vi "MateChecker.vi"(10 "Turn":T1, 11 "Input Squares":T2[][](array[typedef])) -> (3 "Checkmate?":bool)   [LabVIEW 2019]
uses:
  #typedef_DataBase.ctl
  #typedef_SquareType.ctl
  #typedef_Color.ctl
  #typedef_Piece.ctl
  #typedef_PieceType.ctl
  #typedef_SquareLook.ctl
  #typedef_SpecialMoves.ctl
panel:
  out "?":u16[][](array[ring])
  in  "DataBase":T5
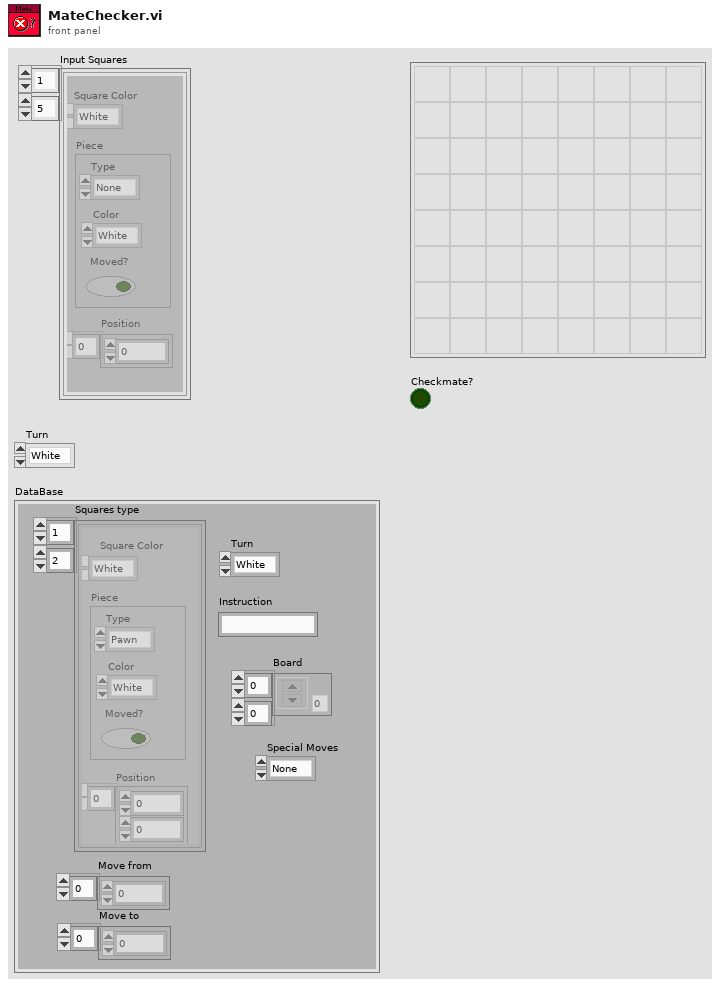
[diagram p1: front panel]
types:
  T1 = typedef "#typedef_Color.ctl" = enum16{"White", "Black"}
  T2 = typedef "#typedef_SquareType.ctl" = cluster{"Square Color":T1, "Position":i32[], "Piece":T3}
  T3 = typedef "#typedef_Piece.ctl" = cluster{"Type":T4, "Color":T1, "Moved?":bool}
  T4 = typedef "#typedef_PieceType.ctl" = enum16{"None", "Pawn", "Knight", "Bishop", "Rook", "Queen", "King"}
  T5 = typedef "#typedef_DataBase.ctl" = cluster{"Squares type":T2[][], "Turn":T1, "Move from":i32[], "Move to":i32[], "Instruction":string, "Board":T6[][], "Special Moves":T7}
  T6 = typedef "#typedef_SquareLook.ctl" = u16
  T7 = typedef "#typedef_SpecialMoves.ctl" = enum16{"None", "Last Square", "Beat in the Passage", "Short Castle", "Long Castle"}
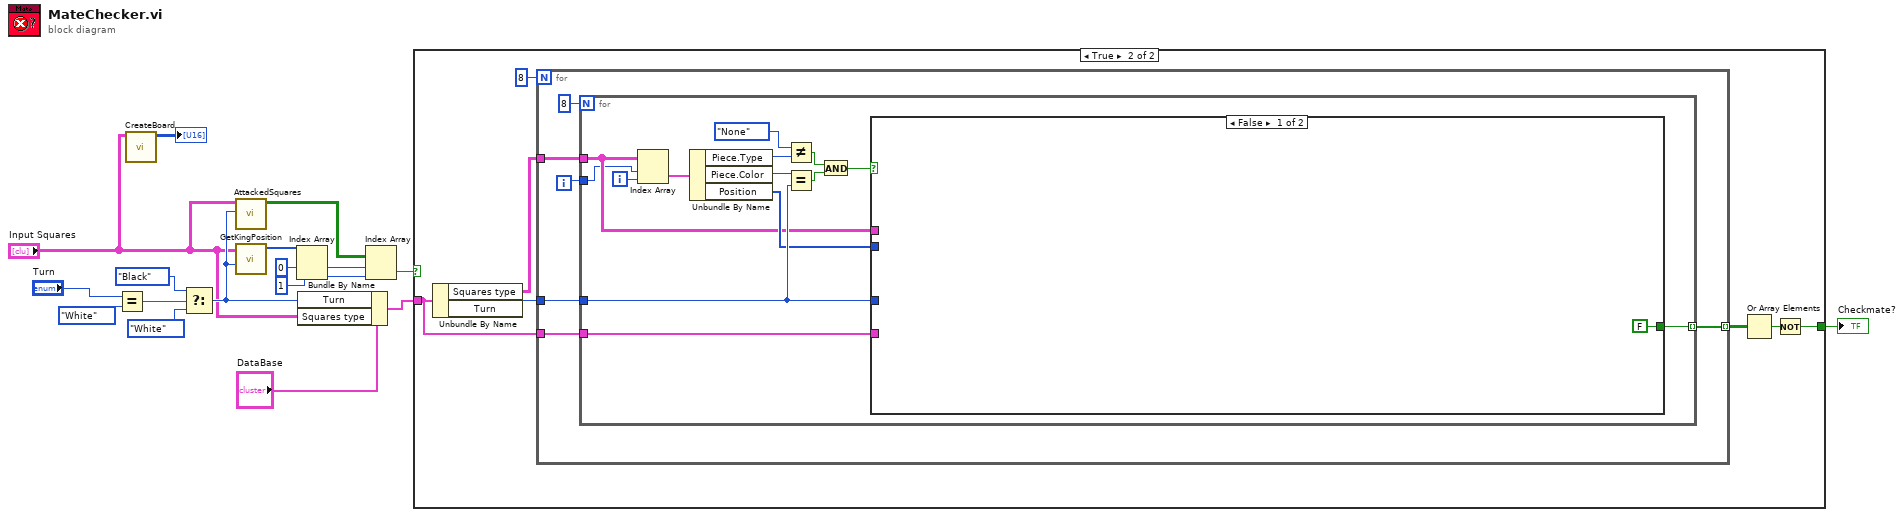
[diagram p0: block diagram]
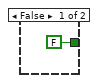
[diagram p2: hidden frame]
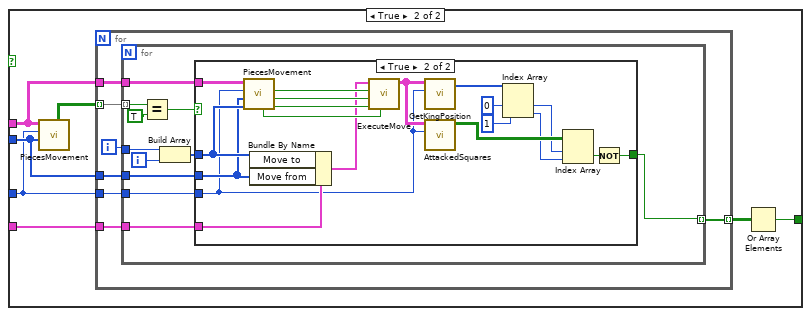
[diagram p3: hidden frame]
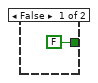
[diagram p4: hidden frame]
diagram:
  n1 = Equal?(x="Turn", y=#typedef_Color."White") -> (x = y?=w3:bool)
  n2 = call "CreateBoard.vi"("Squares type"="Input Squares") -> ("Board"=→"?":u16[][])  [unwired: 10 in]
  n3 = Select(t=#typedef_Color."Black", s=w3, f=#typedef_Color."White" ("y")) -> (s? t:f=w13:T1)
  n4 = call "AttackedSquares.vi"("Turn"=w13, "Input Squares"="Input Squares") -> ("Attacked Squares"=w9:bool[][])  [unwired: 9 in]
  n5 = call "GetKingPosition.vi"("Color"=w13, "Input Squares"="Input Squares") -> ("Position"=w6:i32[])  [unwired: 9 in]
  n6 = Index Array(array=w6, index #1=0 ("index"), index #2=1 ("index")) -> (element #1=w10:i32, element #2=w11:i32)
  n7 = Bundle By Name(cluster="DataBase", "Turn"=w13, "Squares type"="Input Squares") -> (w14:T5)
  n8 = Index Array(array=w9, index (row)=w10, index (col)=w11) -> (element=w12:bool)
  n9 = case shown="True" w12 {
    tunnel: w14 -> [_ w24]
    tunnel: [FALSE w20] -> w15
    frame False {
    }
    frame True {
      n10 = Unbundle By Name(w24) -> ("Squares type"=w26:T2[][], "Turn"=w25:T1)
      n11 = for {
        N: 8 -> [_]
        tunnel: w26 -> [w32]
        tunnel: w25 -> [w31]
        tunnel: w24 -> [w29]
        tunnel: [w27] -> w22 mode=indexing
        i -> [w30]
        n12 = for {
          N: 8 -> [_]
          tunnel: w32 -> [w37]
          tunnel: w31 -> [w40]
          tunnel: w30 -> [w33]
          tunnel: w29 -> [w36]
          tunnel: [w35] -> w27 mode=indexing
          i -> [w34]
          n13 = Index Array(array=w37, index (row)=w33, index (col)=w34) -> (element=w38:T2)
          n14 = Unbundle By Name(w38) -> ("Piece.Type"=w46:T4, "Piece.Color"=w44:T1, "Position"=w39:i32[])
          n15 = Not Equal?(x=#typedef_PieceType."None", y=w46) -> (x != y?=w43:bool)
          n16 = Equal?(x=w44, y=w40) -> (x = y?=w42:bool)
          n17 = And(x=w43, y=w42) -> (x .and. y?=w41:bool)
          n18 = case shown="False" w41 {
            tunnel: w40 -> [_ w51]
            tunnel: w39 -> [_ w52]
            tunnel: w37 -> [_ w53]
            tunnel: w36 -> [_ w50]
            tunnel: [FALSE w48] -> w35
            frame False {
            }
            frame True {
              n19 = call "PiecesMovement.vi"("Move from"=w52, "Turn"=w51, "Input Squares"=w53) -> ("Possible Moves"=w54:bool[][])  [unwired: 3 in, 5 out]
              n20 = for {
                tunnel: w54 -> [w61] mode=indexing
                tunnel: w53 -> [w60]
                tunnel: w52 -> [w58]
                tunnel: w51 -> [w57]
                tunnel: w50 -> [w56]
                tunnel: [w55] -> w49 mode=indexing
                i -> [w59]
                n21 = for {
                  tunnel: w61 -> [w72] mode=indexing
                  tunnel: w60 -> [w69]
                  tunnel: w59 -> [w63]
                  tunnel: w58 -> [w67]
                  tunnel: w57 -> [w66]
                  tunnel: w56 -> [w65]
                  tunnel: [w64] -> w55 mode=indexing
                  i -> [w62]
                  n22 = Equal?(x=w72, y=TRUE) -> (x = y?=w70:bool)
                  n23 = Build Array(w63, w62) -> (w68:i32[])
                  n24 = case shown="True" w70 {
                    tunnel: w69 -> [_ w92]
                    tunnel: w68 -> [_ w86]
                    tunnel: w67 -> [_ w85]
                    tunnel: w66 -> [_ w82]
                    tunnel: w65 -> [_ w87]
                    tunnel: [FALSE w74] -> w64
                    frame False {
                    }
                    frame True {
                      n25 = call "PiecesMovement.vi"("Move to"=w86, "Move from"=w85, "Turn"=w82, "Input Squares"=w92) -> ("Short Castle?"=w91:bool, "Beat in the Passage?"=w90:bool, "Last Square?"=w89:bool, "Long Castle?"=w88:bool)  [unwired: 2 in, 2 out]
                      n26 = Bundle By Name(cluster=w87, "Move to"=w86, "Move from"=w85) -> (w84:T5)
                      n27 = call "ExecuteMove.vi"("Long Castle?"=w88, "Small Castle?"=w91, "In the Passage?"=w90, "Last Square?"=w89, "Input DataBase"=w84) -> ("Output Squares"=w83:T2[][])  [unwired: 6 in]
                      n28 = call "GetKingPosition.vi"("Color"=w82, "Input Squares"=w83) -> ("Position"=w79:i32[])  [unwired: 9 in]
                      n29 = call "AttackedSquares.vi"("Turn"=w82, "Input Squares"=w83) -> ("Attacked Squares"=w78:bool[][])  [unwired: 9 in]
                      n30 = Index Array(array=w79, index #1=0 ("index"), index #2=1 ("index")) -> (element #1=w77:i32, element #2=w76:i32)
                      n31 = Index Array(array=w78, index (row)=w77, index (col)=w76) -> (element=w75:bool)
                      n32 = Not(x=w75) -> (.not. x?=w74:bool)
                    }
                  }
                }
              }
              n33 = Or Array Elements(Boolean array=w49) -> (logical OR=w48:bool)
            }
          }
        }
      }
      n34 = Or Array Elements(Boolean array=w22) -> (logical OR=w21:bool)
      n35 = Not(x=w21) -> (.not. x?=w20:bool)
    }
  }
  "Checkmate?" <- w15
